vi "Servo rotate there and back and show accelerometer values.vi"(8 "Error In":errorcluster) -> (0 "Error Out":errorcluster)   [LabVIEW 2014]
doc: "Tested on:\n - Arduino Nano\n\nRotating servo motor there and back from 0deg to 180deg."
uses:
  LabVIEW-Universal-Transcriptor-ServoLibrary/ServoDatatype.lvclass
  <vilib>/LabVIEW Universal Transcriptor/Arduino MPU6050 Library/Arduino MPU6050.lvlib
  <vilib>/LabVIEW Universal Transcriptor/LabVIEW for Arduino Math Library/Arduino Math.lvlib
panel:
  in  "address":u16(ring)=104 items=["AD0 pin NOT CONNECTED"=104, "AD0 connect to Vcc"=105]
  in  "range":T1(ring)
  in  "scale":T2(ring)
  in  "Servo Pin number":i32=4
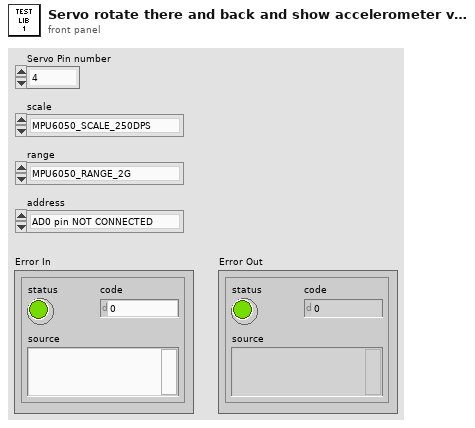
[diagram p1: front panel]
types:
  T1 = enum16{"MPU6050_RANGE_2G", "MPU6050_RANGE_4G", "MPU6050_RANGE_8G", "MPU6050_RANGE_16G"}
  T2 = enum16{"MPU6050_SCALE_250DPS", "MPU6050_SCALE_500DPS", "MPU6050_SCALE_1000DPS", "MPU6050_SCALE_2000DPS"}
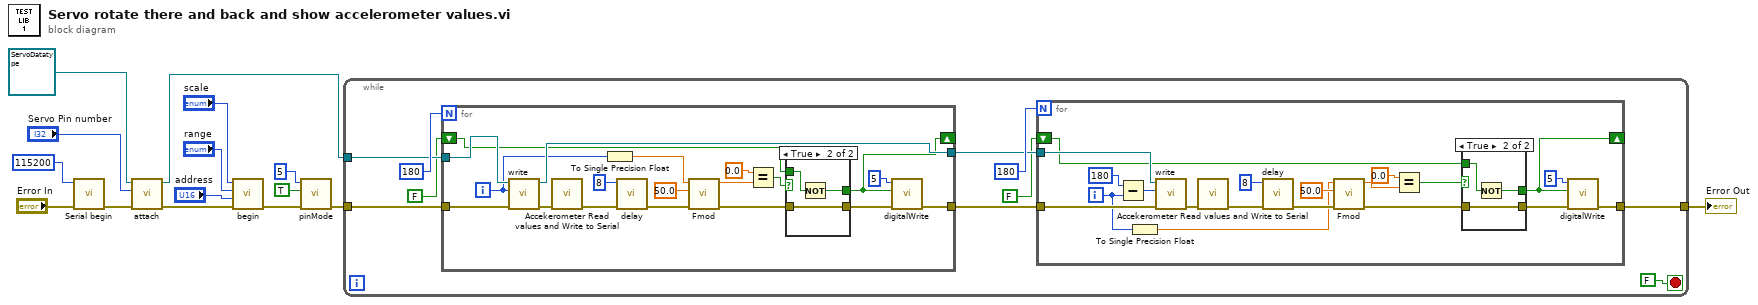
[diagram p0: block diagram]
diagram:
  n1 = call <vilib>:"Serial begin.vi"("Error In"="Error In", "speed (Bd)"=115200) -> ("Error Out"=w6:errorcluster)  [unwired: 9 in]
  n2 = call-dynamic "attach.vi"("error in (no error)"=w6, "pin number"="Servo Pin number", "Servo in"=refnum<class "ServoDatatype.lvclass"> refnum) -> ("error out"=w10:errorcluster, "Servo out"=w9:refnum<class "ServoDatatype.lvclass">)  [unwired: 6 in, 1 out]
  n3 = call <vilib>:"begin.vi"("Error In"=w10, "address"="address", "range"="range", "scale"="scale") -> ("Error Out"=w4:errorcluster)  [unwired: 7 in]
  n4 = call <vilib>:"pinMode.vi"("Error In"=w4, "output?"=TRUE, "pin number"=5) -> ("Error Out"=w3:errorcluster)  [unwired: 8 in]
  n5 = while {
    tunnel: w3 -> [w23]
    tunnel: w9 -> [w24]
    tunnel: [w19] -> w8
    stop <- FALSE stop-if-true
    n6 = for {
      N: 180 -> [_]
      tunnel: w24 -> [w69]
      tunnel: w23 -> [w68]
      tunnel: [w67] -> w21
      tunnel: [w53] -> w17
      shift-right: [w51] -> _
      shift-left: FALSE -> [w55]
      i -> [w62]
      n7 = call-dynamic "write.vi"("error in (no error)"=w68, "value"=w62, "ServoDatatype in"=w69) -> ("error out"=w65:errorcluster, "ServoDatatype out"=w67:refnum<class "ServoDatatype.lvclass">)  [unwired: 7 in]
      n8 = call "Accekerometer Read values and Write to Serial.vi"("error in (no error)"=w65) -> ("error out"=w64:errorcluster)  [unwired: 10 in]
      n9 = To Single Precision Float(number=w62) -> (single precision float=w61:sgl)
      n10 = call <vilib>:"delay.vi"("Error In"=w64, "time (ms)"=8) -> ("Error Out"=w63:errorcluster)  [unwired: 9 in]
      n11 = call <vilib>:"Fmod.vi"("Error In"=w63, "y"=sgl 50.0, "x"=w61) -> ("Error Out"=w59:errorcluster, "fmod(x,y)"=w57:sgl)  [unwired: 7 in]
      n12 = Equal?(x=sgl 0.0, y=w57) -> (x = y?=w58:bool)
      n13 = case shown="True" w58 {
        tunnel: w59 -> [w71 w74]
        tunnel: w55 -> [w70 w73]
        tunnel: [w71 w74] -> w52
        tunnel: [w70 w72] -> w51
        frame False {
        }
        frame True {
          n14 = Not(x=w73) -> (.not. x?=w72:bool)
        }
      }
      n15 = call <vilib>:"digitalWrite.vi"("Error In"=w52, "value"=w51, "pin number"=5) -> ("Error Out"=w53:errorcluster)  [unwired: 8 in]
    }
    n16 = for {
      N: 180 -> [_]
      tunnel: w21 -> [w45]
      tunnel: [w32] -> w19
      tunnel: w17 -> [w40]
      shift-right: [w30] -> _
      shift-left: FALSE -> [w34]
      i -> [w28]
      n17 = Subtract(x=180, y=w28) -> (x-y=w29:i32)
      n18 = To Single Precision Float(number=w28) -> (single precision float=w27:sgl)
      n19 = call-dynamic "write.vi"("error in (no error)"=w40, "value"=w29, "ServoDatatype in"=w45) -> ("error out"=w42:errorcluster)  [unwired: 7 in, 1 out]
      n20 = call "Accekerometer Read values and Write to Serial.vi"("error in (no error)"=w42) -> ("error out"=w41:errorcluster)  [unwired: 10 in]
      n21 = call <vilib>:"delay.vi"("Error In"=w41, "time (ms)"=8) -> ("Error Out"=w36:errorcluster)  [unwired: 9 in]
      n22 = call <vilib>:"Fmod.vi"("Error In"=w36, "y"=sgl 50.0, "x"=w27) -> ("Error Out"=w35:errorcluster, "fmod(x,y)"=w38:sgl)  [unwired: 7 in]
      n23 = Equal?(x=sgl 0.0, y=w38) -> (x = y?=w26:bool)
      n24 = case shown="True" w26 {
        tunnel: [w47 w50] -> w33
        tunnel: w35 -> [w47 w50]
        tunnel: w34 -> [w46 w49]
        tunnel: [w46 w48] -> w30
        frame False {
        }
        frame True {
          n25 = Not(x=w49) -> (.not. x?=w48:bool)
        }
      }
      n26 = call <vilib>:"digitalWrite.vi"("Error In"=w33, "value"=w30, "pin number"=5) -> ("Error Out"=w32:errorcluster)  [unwired: 8 in]
    }
  }
  "Error Out" <- w8
